vi "Test Convert Fixed Time to RFC3339Nano.vi"(8 "error in (no error)":errorcluster) -> (0 "error out":errorcluster)   [LabVIEW 2017, in "UT_LokiJsonFormatter.lvlib"]
doc: "Template for an unit test with caraya in the \"Given, When, Then\" structure from James."
uses:
  UT_LokiJsonFormatter.lvlib
  <vilib>/addons/_JKI Toolkits/Caraya/classes/Assert/Assert Equal Value_Variant.vi
  <vilib>/addons/_JKI Toolkits/Caraya/classes/Test/Test.lvclass
  <vilib>/addons/_JKI Toolkits/Caraya/classes/Assert/Assert.lvclass
  Source/HSE-Logger/Formatter/LokiJsonFormatter/LokiJsonFormatter.lvclass
panel:
  # "Connector Pane"
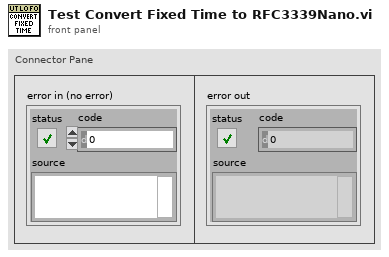
[diagram p1: front panel]
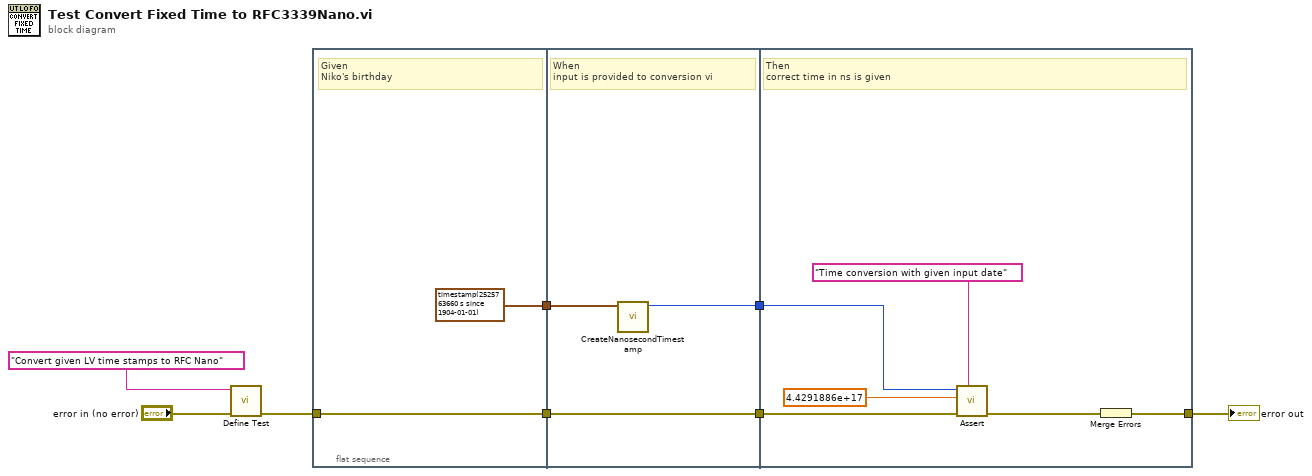
[diagram p0: block diagram]
diagram:
  n1 = call <vilib>:"Define Test.vi"("error in (no error)"="error in (no error)", "Label (VI Title)"="Convert given LV time stamps to RFC Nano") -> ("error out"=w5:errorcluster)  [unwired: 8 in, 1 out]
  n2 = flat-sequence {
    tunnel: w5 -> [w10]
    tunnel: [w10] -> w8
    tunnel: [timestamp(2525763660 s since 1904-01-01) ("current time")] -> w2
    tunnel: w8 -> [w13]
    tunnel: [w13] -> w3
    tunnel: w2 -> [w12]
    tunnel: [w11] -> w1
    tunnel: [w18] -> w7
    tunnel: w3 -> [w17]
    tunnel: w1 -> [w14]
    frame #0 {
      # "Given\nNiko's birthday"
    }
    frame #1 {
      # "When\ninput is provided to conversion vi"
      n3 = call "CreateNanosecondTimestamp.vi"("current time"=w12) -> ("Time in RFC3339Nano"=w11:i64)  [unwired: 9 in, 1 out]
    }
    frame #2 {
      # "Then\ncorrect time in ns is given"
      n4 = call-poly <vilib>:"Assert.vi"("Label"="Time conversion with given input date", "error in (no error)"=w17, "Actual"=4.4291886e+17, "Expected"=w14) -> ("error out"=w19:errorcluster)  [unwired: 6 in, 1 out]
      n5 = Merge Errors(w19) -> (w18:errorcluster)
    }
  }
  "error out" <- w7
